vi "Set Auxiliary Amplifier.vi"(8 "error in (no error)":errorcluster, 9 "Current Boost (0: None)":u32(ring) items=["None", "5725A", "5220A"], 10 "Voltage Boost (0: None)":u32(ring) items=["None", "5725A", "5205A", "5215A"], 11 "VISA resource name":refnum<visa-resource-name>) -> (0 "error out":errorcluster, 3 "VISA resource name out":refnum<visa-resource-name>)   [LabVIEW 2011, in "Fluke 5XXX Series Multicalibrators.lvlib"]
doc: "This VI selects the accessory amplifiers for current and voltage boost. The setting of this VI remains even after the power is turned off.\n\nNotes:\n\n(1) This VI is available only for instrument models 5700A and 5720A.\n\n(2) This VI does not take effect until the auxiliary amplifier is active."
uses:
  Fluke 5XXX Series Multicalibrators.lvlib
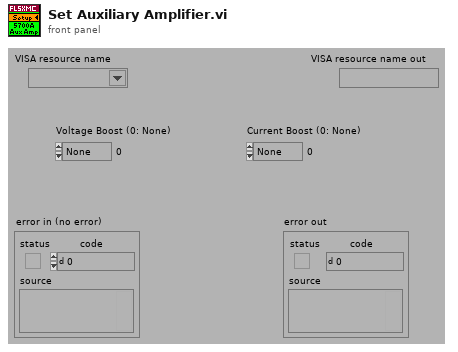
[diagram p1: front panel]
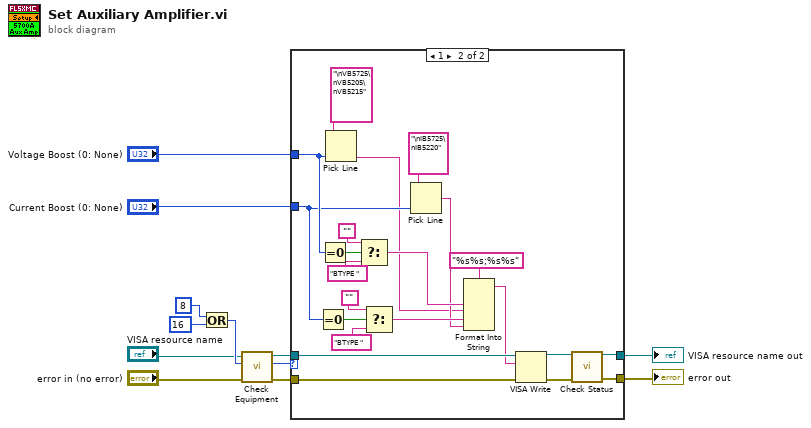
[diagram p0: block diagram]
diagram:
  n1 = Or(x=8 ("Numeric"), y=16 ("Numeric")) -> (x .or. y?=w9:i32)
  n2 = call "Check Equipment.vi"("error in (no error)"="error in (no error)", "Bit Mask"=w9, "VISA resource name"="VISA resource name") -> ("error out"=w12:errorcluster, "Present?"=w11:u32, "VISA resource name out"=w10:refnum<visa-resource-name>)  [unwired: 6 in]
  n3 = case shown="1" w11 {
    tunnel: [w13 w30] -> w4
    tunnel: w12 -> [w14 w35]
    tunnel: w10 -> [w13 w34]
    tunnel: [w14 w33] -> w3
    tunnel: "Current Boost (0: None)" -> [_ w26]
    tunnel: "Voltage Boost (0: None)" -> [_ w27]
    frame 0, Default {
    }
    frame 1 {
      n4 = Equal To 0?(x=w26) -> (x = 0?=w25:bool)
      n5 = Equal To 0?(x=w27) -> (x = 0?=w24:bool)
      n6 = Pick Line(multi-line string="\nVB5725\nVB5205\nVB5215", line index=w27) -> (output string=w16:string)  [unwired: 1 in]
      n7 = Select(t="", s=w24, f="BTYPE " ("Reset Command")) -> (s? t:f=w19:string)
      n8 = Select(t="", s=w25, f="BTYPE " ("Reset Command")) -> (s? t:f=w18:string)
      n9 = Pick Line(multi-line string="\nIB5725\nIB5220", line index=w26) -> (output string=w17:string)  [unwired: 1 in]
      n10 = Format Into String(format string="%s%s;%s%s" ("Reset Command"), w19, w16, w18, w17) -> (resulting string=w15:string)  [unwired: 2 in, 1 out]
      n11 = VISA Write(VISA resource name=w34, write buffer=w15, error in (no error)=w35) -> (VISA resource name out=w31:refnum<visa-resource-name>, error out=w32:errorcluster)  [unwired: 1 out]
      n12 = call "Check Status.vi"("VISA resource name"=w31, "error in (no error)"=w32) -> ("VISA resource name out"=w30:refnum<visa-resource-name>, "error out"=w33:errorcluster)  [unwired: 12 in]
    }
  }
  "VISA resource name out" <- w4
  "error out" <- w3
